vi "Write ASCII Message.vi"(8 "error in":errorcluster, 10 "Message":string, 11 "VISA resource in":refnum<visa-resource-name>) -> (0 "error out":errorcluster, 3 "VISA resource out":refnum<visa-resource-name>)   [LabVIEW 2019]
doc: "Builds up the ASCII message and then sends it through the serial port."
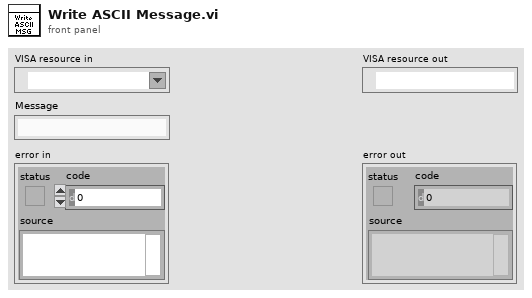
[diagram p1: front panel]
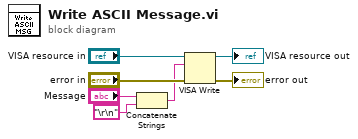
[diagram p0: block diagram]
diagram:
  n1 = Concatenate Strings("Message", "\r\n") -> (w2:string)
  n2 = VISA Write(VISA resource name="VISA resource in", write buffer=w2, error in (no error)="error in") -> (VISA resource name out=→"VISA resource out":refnum<visa-resource-name>, error out=→"error out":errorcluster)  [unwired: 1 out]
